vi "get_paths.vi"() -> (14 "html path":path, 15 "LV web ui path":path)   [LabVIEW 2020, in "simple_html_chat_ui.lvclass"]
uses:
  simple_html_chat_ui.lvclass
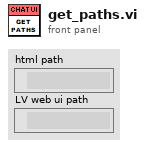
[diagram p1: front panel]
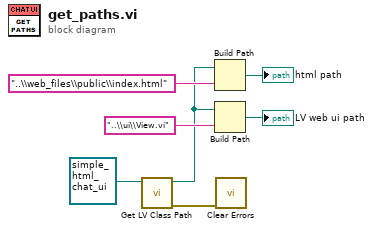
[diagram p0: block diagram]
diagram:
  n1 = call <vilib>:"Get LV Class Path.vi"("object"=refnum<class "simple_html_chat_ui.lvclass"> refnum ("simple_html_chat_ui in")) -> ("error out"=w3:errorcluster, "class path"=w4:path)  [unwired: 9 in]
  n2 = Build Path(base path=w4, name or relative path="..\\web_files\\public\\index.html") -> (appended path=→"html path":path)
  n3 = Build Path(base path=w4, name or relative path="..\\ui\\View.vi") -> (appended path=→"LV web ui path":path)
  n4 = call <vilib>:"Clear Errors.vi"("error in (no error)"=w3) -> ()  [unwired: 5 in, 2 out]
